vi "wdt.vi"() -> ()   [LabVIEW 2021]
panel:
  in  "wdt":waveform(dbl)
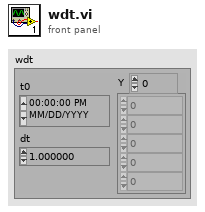
[diagram p1: front panel]
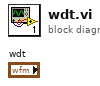
[diagram p0: block diagram]
diagram:
